vi "SimulateTempeartures.vi"() -> (3 "Simulated Temperatures":dbl[][](array[numeric]))   [LabVIEW 2012]
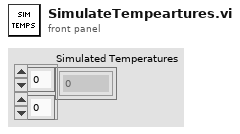
[diagram p1: front panel]
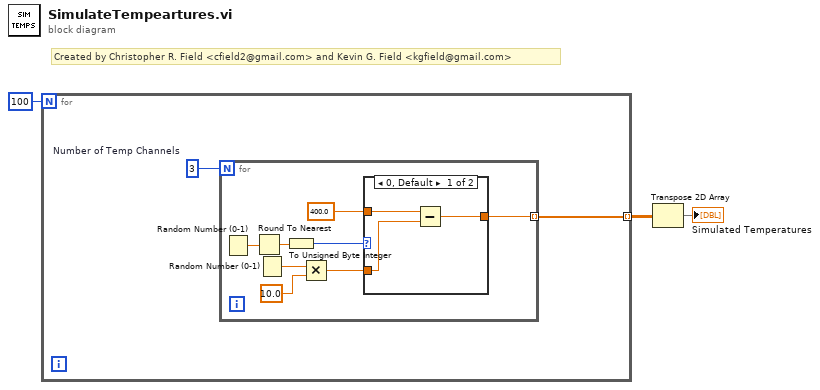
[diagram p0: block diagram]
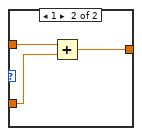
[diagram p2: hidden frame]
diagram:
  # "Created by Christopher R. Field <cfield2@gmail.com> and Kevin G. Field <kgfield@gmail.com>"
  n1 = for {
    N: 100 -> [_]
    tunnel: [w4] -> w2 mode=indexing
    w5 = 3  # Number of Temp Channels
    n2 = for {
      N: w5 -> [_]
      tunnel: [w9] -> w4 mode=indexing
      n3 = Random Number (0-1)() -> (number: 0 to 1=w13:dbl)
      n4 = Round To Nearest(number=w13) -> (nearest integer value=w12:dbl)
      n5 = Random Number (0-1)() -> (number: 0 to 1=w8:dbl)
      n6 = To Unsigned Byte Integer(number=w12) -> (unsigned 8bit integer=w11:u8)
      n7 = Multiply(x=w8, y=10.0) -> (x*y=w7:dbl)
      n8 = case shown="0, Default" w11 {
        tunnel: 400.0 -> [w16 w19]
        tunnel: [w15 w18] -> w9
        tunnel: w7 -> [w14 w17]
        frame 0, Default {
          n9 = Subtract(x=w16, y=w14) -> (x-y=w15:dbl)
        }
        frame 1 {
          n10 = Add(x=w19, y=w17) -> (x+y=w18:dbl)
        }
      }
    }
  }
  n11 = Transpose 2D Array(2D array=w2) -> (transposed array=→"Simulated Temperatures":dbl[][])
